vi "DSF.Shared.Configuration.Framework.Set Plugin Configurations.vi"(8 "error in (no error)":errorcluster, 10 "Plugin Configurations":refnum<class "DSF.Shared.Configuration.Plugin.lvclass">[](array[class]), 11 "Framework Configuration in":refnum<class "DSF.Shared.Configuration.Framework.lvclass">) -> (0 "error out":errorcluster, 3 "Framework Configuration out":refnum<class "DSF.Shared.Configuration.Framework.lvclass">)   [LabVIEW 2016, in "DSF.Shared.lvlib" / "DSF.Shared.Configuration.Framework.lvclass"]
uses:
  DSF.Shared.Configuration.Framework.lvclass
  Plugin/DSF.Shared.Configuration.Plugin.lvclass
  DSF.Shared.Configuration.Framework.lvclass/DSF.Shared.Configuration.Framework.ctl
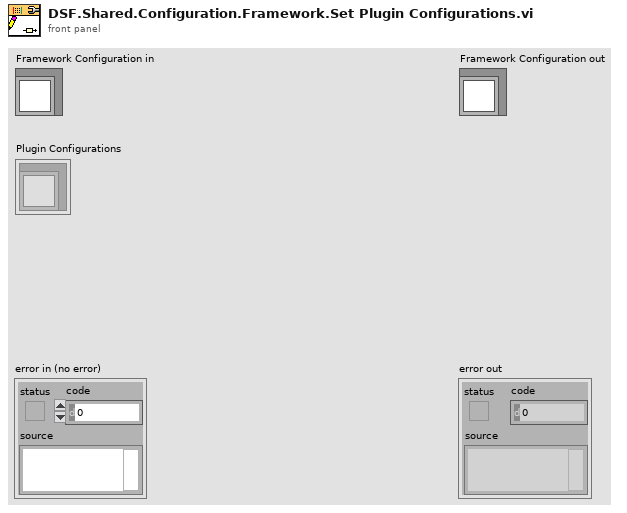
[diagram p1: front panel]
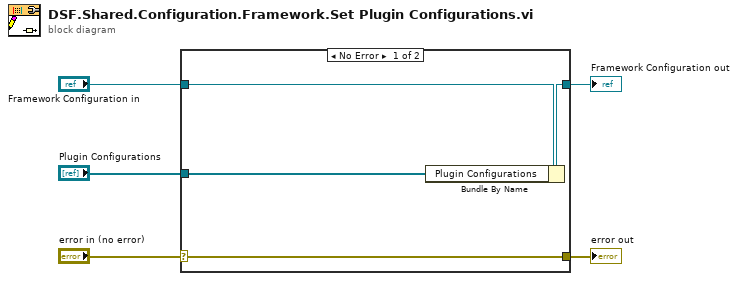
[diagram p0: block diagram]
diagram:
  n1 = case shown="No Error" "error in (no error)" {
    selector: "error in (no error)" -> [w9 w10]
    tunnel: [w9 w10] -> w4
    tunnel: [w7 w11] -> w2
    tunnel: "Framework Configuration in" -> [w8 w11]
    tunnel: "Plugin Configurations" -> [w6 _]
    frame No Error {
      n2 = Bundle By Name(cluster=w8, "Plugin Configurations"=w6) -> (w7:refnum<class "DSF.Shared.Configuration.Framework.lvclass">)
    }
    frame Error {
    }
  }
  "error out" <- w4
  "Framework Configuration out" <- w2
